vi "Fetch Multiple Record Single Channel (4xI16).vi"(7 "Timeout (s)":i32=5, 8 "error in":errorcluster, 10 "Records to Fetch":i64, 11 "FPGA VI Reference In":refnum<k20>) -> (0 "error out":errorcluster, 2 "Acquired Data":i16[][](array[numeric]), 3 "FPGA VI Reference Out":refnum<k20>, 4 "Elements Remaining":u32)   [LabVIEW 2012]
uses:
  <vilib>/Utility/error.llb/Error Cluster From Error Code.vi
  <vilib>/rvi/errors/niLvFpgaAdjustHostInterfaceError.vi
  <vilib>/rvi/interface/nirviReadWriteControl/nirviReadWriteControl.xnode
  NiFpgaLv.dll
  <vilib>/rvi/interface/Simulation/niFpgaSimulationCallBeginRW.vi
panel:
  out "Data Acquired":i16[](array[numeric])
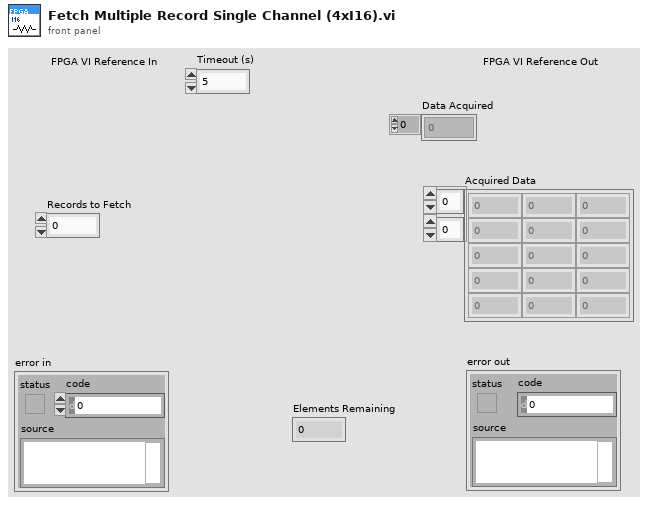
[diagram p1: front panel]
types:
  T1 = cluster{"Load Record Parameters?":bool, "Pre Trigger Samples":u16, "Samples per Record":u16, "Trigger Hold Off":u16, "Record Count":u16}
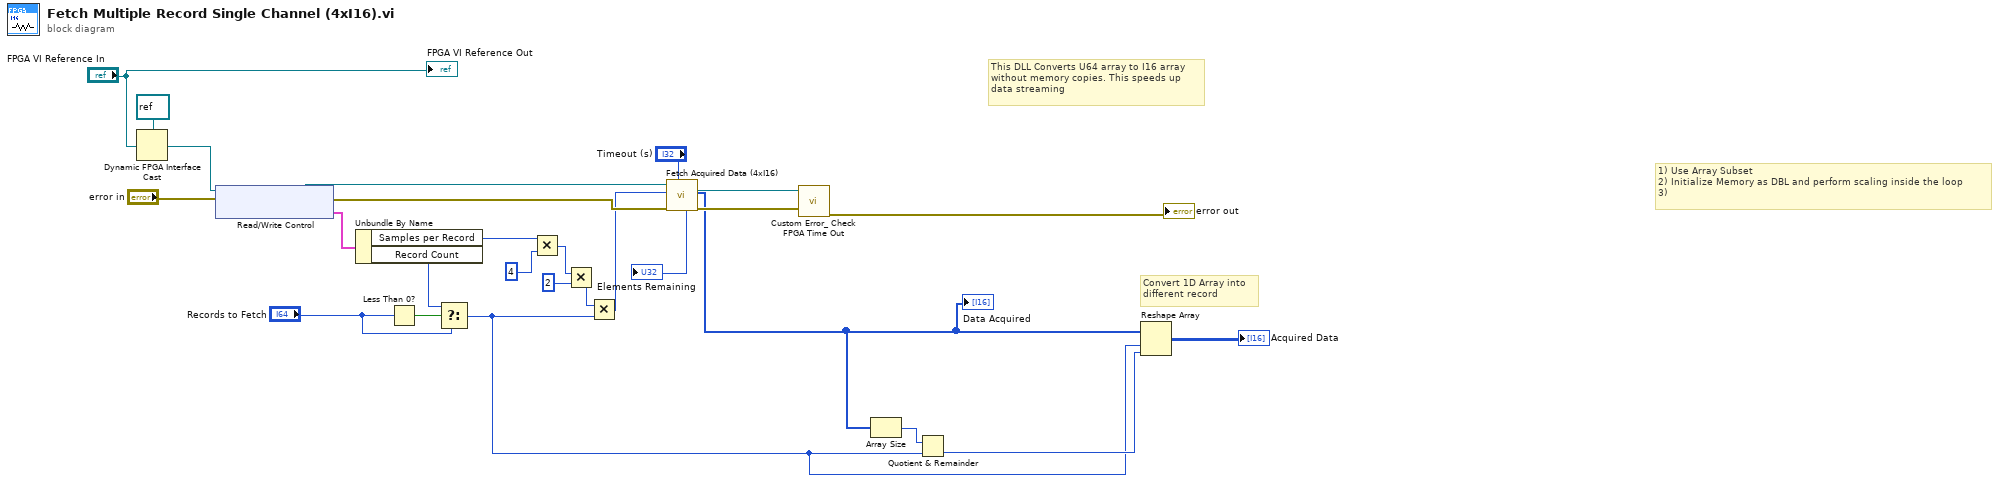
[diagram p0: block diagram]
diagram:
  # "This DLL Converts U64 array to I16 array \nwithout memory copies. This speeds up \ndata streaming"
  # "Convert 1D Array into\ndifferent record"
  # "1) Use Array Subset\n2) Initialize Memory as DBL and perform scaling inside the loop\n3)"
  n1 = Dynamic FPGA Interface Cast(Session In=refnum<k20> refnum ("Type"), Type="FPGA VI Reference In") -> (Session Out=w23:refnum<k20>)
  n2 = xnode "Read/Write Control"("FPGA VI Reference In"=w23, "error in"="error in") -> ("FPGA VI Reference Out"=w18:refnum<k20>, "error out"=w17:errorcluster, "Record Parameters"=w22:T1)
  n3 = Unbundle By Name(w22) -> ("Samples per Record"=w7:u16, "Record Count"=w20:u16)
  n4 = Less Than 0?(x="Records to Fetch") -> (x < 0?=w21:bool)
  n5 = Select(t=w20, s=w21, f="Records to Fetch") -> (s? t:f=w8:i64)
  n6 = Multiply(x=w7, y=u64 4) -> (x*y=w3:u64)
  n7 = Multiply(x=w3, y=u64 2) -> (x*y=w1:u64)
  n8 = Multiply(x=w1, y=w8) -> (x*y=w12:u64)
  n9 = call <userlib>:"Fetch Acquired Data (4xI16).vi"("Timeout (s)"="Timeout (s)", "error out"=w17, "Samples"=w12, "FPGA Ref In"=w18) -> ("error out"=w13:errorcluster, "Data"=w5:i16[], "FPGA RefOut"=w14:refnum<k20>, "Elements Remaining"=→"Elements Remaining":u32)  [unwired: 4 in]
  "Data Acquired" <- w5
  n10 = call <userlib>:"Custom Error_ Check FPGA Time Out.vi"("error in"=w13, "FPGA VI Reference In"=w14) -> ("error out"=→"error out":errorcluster)  [unwired: 8 in, 1 out]
  n11 = Array Size(array=w5) -> (size(s)=w6:i32)
  n12 = Quotient & Remainder(x=w6, y=w8) -> (floor(x/y)=w9:i64)  [unwired: 1 out]
  n13 = Reshape Array(w5, w8, w9) -> (→"Acquired Data":i16[][])
  "FPGA VI Reference Out" <- "FPGA VI Reference In"
